vi "GLdrv_SCAL_SET.vi"(0 "Connection ID":T2, 5 "CH":i32=1 min=1, 7 "Scale":T1, 11 "error in (no error)":errorcluster, 13 "Query(f)":bool) -> (4 "Connection ID Out":T2, 8 "Scale out":T1, 15 "error out":errorcluster)   [LabVIEW 2017, in "GL860_Driver.lvlib"]
doc: "スケーリングの変換値の設定・参照\n測定上限値：　測定値側（入力側）の上限値を物理値で設定します\n測定下限値：　測定値側（入力側）の下限値を物理値で設定します\n”測定値単位”：　測定値側の物理単位を設定します（省略可能）\nEU上限値：　変換値側の上限値を物理値で設定します\nEU下限値：　変換値側の下限値を物理値で設定します\n”EU単位”：　変換値側の物理単位を設定します\n※EU上限値/下限値の小数点位置が小数点以下4桁まで設定に反映\nされます。また、上限値と下限値の小数点位置は同じにしてください。\n※温度時は測定上限値/下限値、EU上限値/下限値のそれぞれを同\nじ値に設定します。\n例）　:SCAL:CH4:SET 200.00,-200.00,”V”,50.00,-50.00,”hPa” (アナ\nログ入力CH4のスケーリングを200V,-200Vを50.00hPa,-50.00hPaに\n単位変換します。)"
uses:
  GL860_Driver.lvlib
  ConnectionID.ctl
  GLdrv_RW.ctl
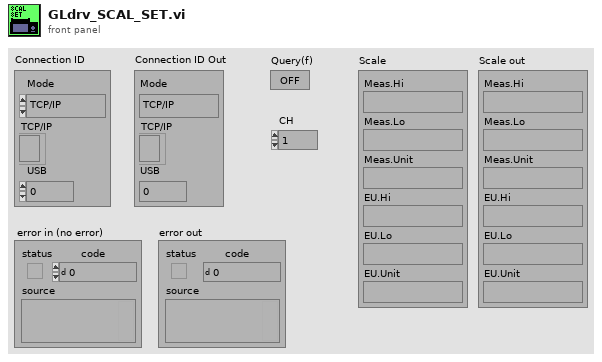
[diagram p1: front panel]
types:
  T1 = cluster{"Meas.Hi":string, "Meas.Lo":string, "Meas.Unit":string, "EU.Hi":string, "EU.Lo":string, "EU.Unit":string}
  T2 = typedef "ConnectionID.ctl" = cluster{"Mode":enum16{"TCP/IP", "USB"}, "TCP/IP":refnum<k5>, "USB":i32}
  T3 = typedef "GLdrv_RW.ctl" = enum16{"Auto", "Read", "Write", "Buffer"}
  T4 = cluster{"[0]":string, "[1]":string, "[2]":string, "[3]":string, "[4]":string, "[5]":string}
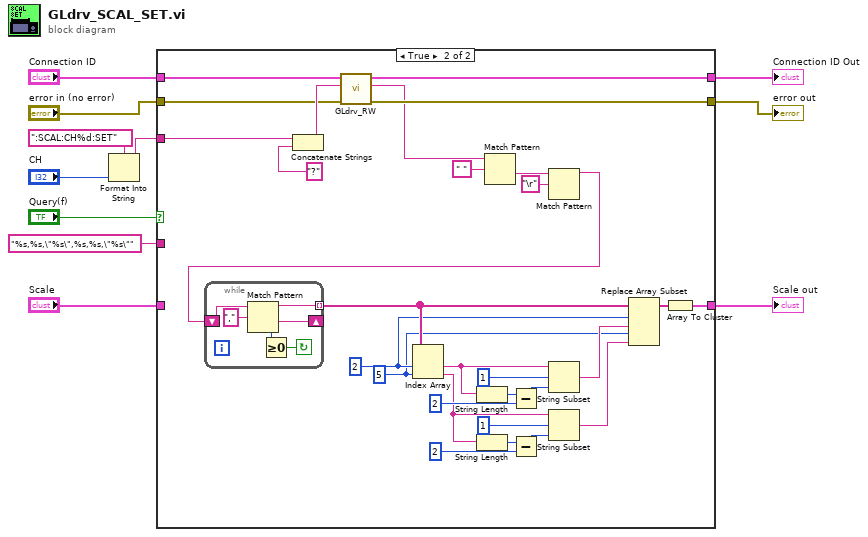
[diagram p0: block diagram]
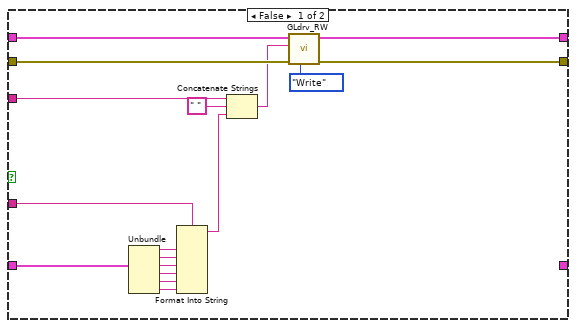
[diagram p2: hidden frame]
diagram:
  n1 = Format Into String(format string=":SCAL:CH%d:SET" ("Command"), "CH") -> (resulting string=w5:string)  [unwired: 2 in, 1 out]
  n2 = case shown="TRUE" "Query(f)" {
    tunnel: w5 -> [w28 w57]
    tunnel: [w23 w51] -> w11
    tunnel: [w25 w54] -> w10
    tunnel: "Connection ID" -> [w26 w55]
    tunnel: "error in (no error)" -> [w24 w52]
    tunnel: "%s,%s,\"%s\",%s,%s,\"%s\"" ("Param") -> [w19 _]
    tunnel: "Scale" -> [w18 _]
    tunnel: [_ w50] -> w2
    frame False {
      n3 = Unbundle(w18) -> ("Meas.Hi"=w17:string, "Meas.Lo"=w16:string, "Meas.Unit"=w15:string, "EU.Hi"=w14:string, "EU.Lo"=w13:string, "EU.Unit"=w12:string)
      n4 = Format Into String(format string=w19, w17, w16, w15, w14, w13, w12) -> (resulting string=w20:string)  [unwired: 2 in, 1 out]
      n5 = Concatenate Strings(w28, " " ("string"), w20) -> (w22:string)
      n6 = call "GLdrv_RW.vi"("Mode(read)"=GLdrv_RW."Write", "error in (no error)"=w24, "data in"=w22, "Connection ID"=w26) -> ("error out"=w23:errorcluster, "Connection ID Out"=w25:T2)  [unwired: 3 in, 3 out]
    }
    frame True {
      w31 = 2 ("index")
      w30 = 5 ("index")
      n7 = Concatenate Strings(w57, "?" ("string")) -> (w53:string)
      n8 = call "GLdrv_RW.vi"("error in (no error)"=w52, "data in"=w53, "Connection ID"=w55) -> ("error out"=w51:errorcluster, "data out"=w29:string, "Connection ID Out"=w54:T2)  [unwired: 4 in, 2 out]
      n9 = Match Pattern(string=w29, regular expression=" " ("search string/char (-)")) -> (after substring=w47:string)  [unwired: 4 out]
      n10 = Match Pattern(string=w47, regular expression="\r") -> (before substring=w46:string)  [unwired: 4 out]
      n11 = while {
        shift-right: [w62] -> _
        shift-left: w46 -> [w61]
        tunnel: [w59] -> w45 mode=indexing
        stop <- w58 continue-if-true
        n12 = Match Pattern(string=w61, regular expression=",") -> (before substring=w59:string, after substring=w62:string, offset past match=w63:i32)  [unwired: 2 out]
        n13 = Greater Or Equal To 0?(x=w63) -> (x >= 0?=w58:bool)
      }
      n14 = Index Array(array=w45, index #1=w31, index #2=w30) -> (element #1=w39:string, element #2=w34:string)
      n15 = String Length(string=w39) -> (length=w42:i32)
      n16 = String Length(string=w34) -> (length=w36:i32)
      n17 = Subtract(x=w42, y=2) -> (x-y=w41:i32)
      n18 = Subtract(x=w36, y=2) -> (x-y=w37:i32)
      n19 = String Subset(string=w39, offset (0)=1, length (rest)=w41) -> (substring=w33:string)
      n20 = String Subset(string=w34, offset (0)=1, length (rest)=w37) -> (substring=w32:string)
      n21 = Replace Array Subset(array=w45, new element #1=w33, index #1=w31, new element #2=w32, index #2=w30) -> (w44:string[])
      n22 = Array To Cluster(array=w44) -> (cluster=w50:T4)
    }
  }
  "Connection ID Out" <- w10
  "error out" <- w11
  "Scale out" <- w2
